vi "DANTE close.vi"() -> (0 "error out":errorcluster, 2 "identifier out":string, 3 "function return":bool)   [LabVIEW 2015]
uses:
  XGL_DPP.lvlib
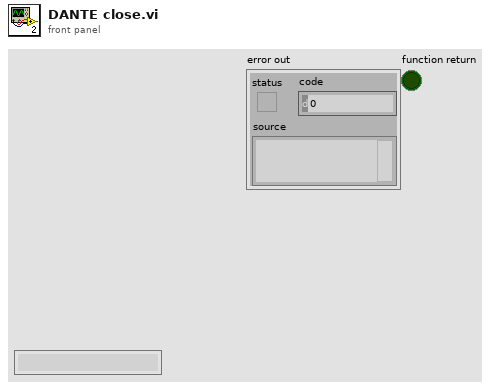
[diagram p1: front panel]
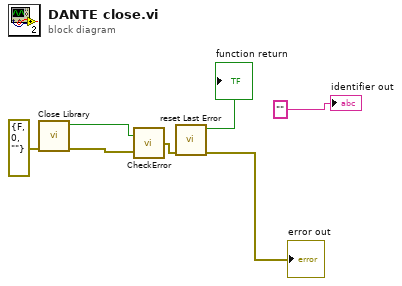
[diagram p0: block diagram]
diagram:
  n1 = call "Close Library.vi"("error in (no error)"=errorcluster {"status"=FALSE, "code"=0, "source"=""}) -> ("error out"=w6:errorcluster, "function return"=w5:bool)  [unwired: 9 in]
  n2 = call "CheckError.vi"("error in (no error)"=w6, "ret_val"=w5) -> ("error out"=w7:errorcluster)
  n3 = call "reset Last Error.vi"("error in (no error)"=w7) -> ("error out"=→"error out":errorcluster, "function return"=→"function return":bool)  [unwired: 9 in]
  "identifier out" <- "" ("identifier out")
